vi "Encoders.vi"(10 "Reset":bool=TRUE, 11 "Enum":enum16{"Start", "Run", "End"}(ring)) -> (0 "Turning Speed":dbl, 1 "Linear Speed":dbl, 2 "RSpeed":dbl, 3 "LSpeed":dbl, 4 "LDistance":dbl, 5 "RDistance":dbl)   [LabVIEW 2014]
uses:
  <vilib>/Rock Robotics/SystemInterfaces/DIO/FPGA_DIOChannel.ctl
  <vilib>/Rock Robotics/WPI/Counter/WPI_CounterDigitalInputToDigitalSource.vi
  <vilib>/Rock Robotics/Network Tables/SD Write Number.vi
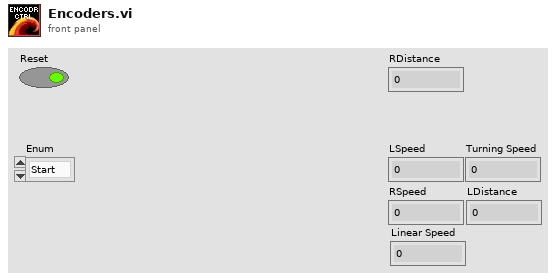
[diagram p1: front panel]
types:
  T1 = typedef "FPGA_DIOChannel.ctl" = enum8{"DIO 0", "DIO 1", "DIO 2", "DIO 3", "DIO 4", "DIO 5", "DIO 6", "DIO 7", "DIO 8", "DIO 9", "DIO MXP 0", "DIO MXP 1", "DIO MXP 2", "DIO MXP 3", "DIO MXP 4", "DIO MXP 5", "DIO MXP 6", "DIO MXP 7", "DIO MXP 8", "DIO MXP 9", "DIO MXP 10", "DIO MXP 11", "DIO MXP 12", "DIO MXP 13", "DIO MXP 14", "DIO MXP 15", "Invalid"}
  T2 = typedef "WPI_DigitalInputDevRef.ctl" = cluster{"DevStatus":errorcluster, "DIO Channel":T1, "Controller":T3}
  T3 = typedef "FPGA_TypedefDigitalModule.ctl" = enum16{"Controller 1"}
  T4 = typedef "FPGA_CounterEncoderSourceConvertionLVSourceType.ctl" = cluster{"DevStatus":errorcluster, "AnalogTriggerMode?":bool, "DigitalMode":cluster{"Controller":T3, "DIO Channel":T5}, "AnalogTriggerMode":cluster{"AnalogTriggerIndex":T6, "OutputType":T7}}
  T5 = typedef "FPGA_DIODigitalSourceChannel.ctl" = enum8{"DIO 0", "DIO 1", "DIO 2", "DIO 3", "DIO 4", "DIO 5", "DIO 6", "DIO 7", "DIO 8", "DIO 9", "DIO MXP 0", "DIO MXP 1", "DIO MXP 2", "DIO MXP 3", "DIO MXP 4", "DIO MXP 5", "DIO MXP 6", "DIO MXP 7", "DIO MXP 8", "DIO MXP 9", "DIO MXP 10", "DIO MXP 11", "DIO MXP 12", "DIO MXP 13", "DIO MXP 14", "DIO MXP 15", "Disabled"}
  T6 = typedef "FPGA_AnalogTriggerIndex.ctl" = enum8{"Trig 0", "Trig 1", "Trig 2", "Trig 3", "Trig 4", "Trig 5", "Trig 6", "Trig 7", "Invalid"}
  T7 = typedef "FPGA_AnalogTriggerOutType.ctl" = enum16{"InWindow", "TriggerState", "Rising", "Falling"}
  T8 = typedef "WPI_EncoderDevRef.ctl" = cluster{"DevStatus":errorcluster, "EncoderIndex":T9, "CounterIndex":T10, "DistancePerCount":dbl, "Decoding Type":T11}
  T9 = typedef "FPGA_EncoderIdx.ctl" = enum8{"Enc 0", "Enc 1", "Enc 2", "Enc 3", "Enc 4", "Enc 5", "Enc 6", "Enc 7", "Invalid"}
  T10 = typedef "FPGA_CounterCtrSystemIndex.ctl" = enum8{"Ctr 0", "Ctr 1", "Ctr 2", "Ctr 3", "Ctr 4", "Ctr 5", "Ctr 6", "Ctr 7", "Invalid"}
  T11 = typedef "WPI_EncoderType.ctl" = enum16{"1x", "2x", "4x"}
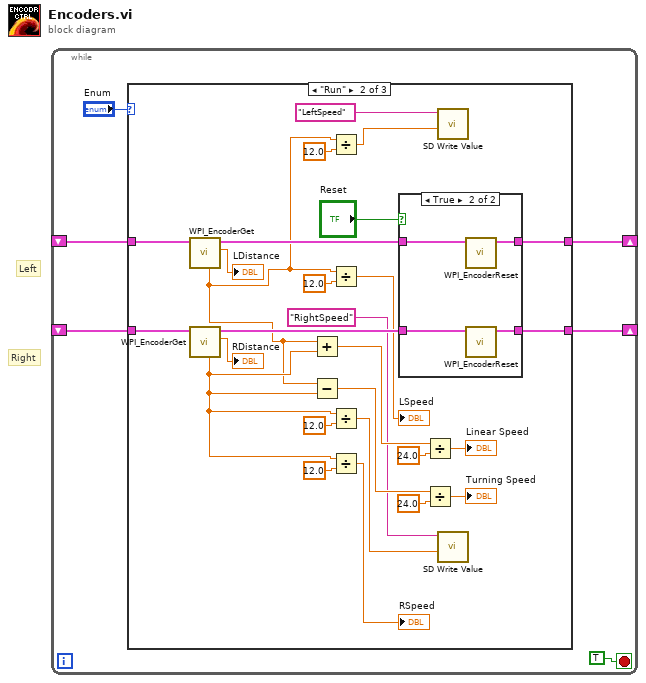
[diagram p0: block diagram]
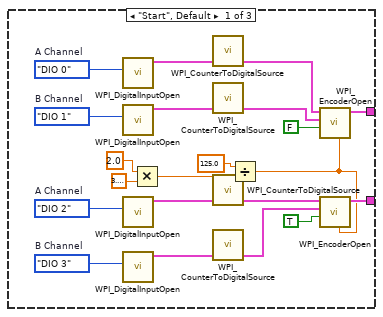
[diagram p2: hidden frame]
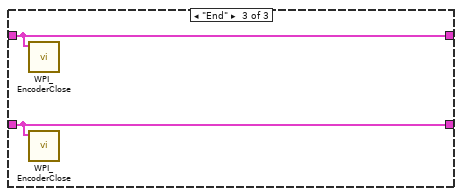
[diagram p4: hidden frame]
diagram:
  # "Right"
  # "Left"
  n1 = while {
    shift-right: [w4] -> _
    shift-left: _ -> [w2]
    shift-right: [w3] -> _
    shift-left: _ -> [w1]
    stop <- TRUE stop-if-true
    n2 = case shown="\"Run\"" "Enum" {
      tunnel: [w15 w44 w61] -> w4
      tunnel: [w14 w42 w62] -> w3
      tunnel: w2 -> [_ w54 w61]
      tunnel: w1 -> [_ w53 w62]
      frame "Start", Default {
        w21 = FPGA_DIOChannel."DIO 3"  # B Channel
        w20 = FPGA_DIOChannel."DIO 2"  # A Channel
        w27 = FPGA_DIOChannel."DIO 1"  # B Channel
        w26 = FPGA_DIOChannel."DIO 0"  # A Channel
        n3 = call <vilib>:"WPI_DigitalInputOpen.vi"("DIO Channel"=w26) -> ("DigitalInputDevRef"=w23:T2)  [unwired: 2 in, 8 out]
        n4 = call <vilib>:"WPI_DigitalInputOpen.vi"("DIO Channel"=w27) -> ("DigitalInputDevRef"=w24:T2)  [unwired: 2 in, 8 out]
        n5 = call <vilib>:"WPI_DigitalInputOpen.vi"("DIO Channel"=w20) -> ("DigitalInputDevRef"=w17:T2)  [unwired: 2 in, 8 out]
        n6 = call <vilib>:"WPI_DigitalInputOpen.vi"("DIO Channel"=w21) -> ("DigitalInputDevRef"=w18:T2)  [unwired: 2 in, 8 out]
        n7 = Multiply(x=2.0, y=3.141592653589793) -> (x*y=w9:dbl)
        n8 = call-poly <vilib>:"WPI_CounterToDigitalSource.vi"("DigitalInputDevRef"=w23) -> ("Digital Source"=w22:T4)  [unwired: 6 out]
        n9 = call-poly <vilib>:"WPI_CounterToDigitalSource.vi"("DigitalInputDevRef"=w24) -> ("Digital Source"=w25:T4)  [unwired: 6 out]
        n10 = call-poly <vilib>:"WPI_CounterToDigitalSource.vi"("DigitalInputDevRef"=w17) -> ("Digital Source"=w16:T4)  [unwired: 6 out]
        n11 = call-poly <vilib>:"WPI_CounterToDigitalSource.vi"("DigitalInputDevRef"=w18) -> ("Digital Source"=w19:T4)  [unwired: 6 out]
        n12 = Divide(x=125.0, y=w9) -> (x/y=w7:dbl)
        n13 = call <vilib>:"WPI_EncoderOpen.vi"("DistancePerCount"=w7, "Invert Direction (False)"=FALSE, "BSource"=w25, "ASource"=w22) -> ("EncoderDevRef"=w15:T8)  [unwired: 4 in, 3 out]
        n14 = call <vilib>:"WPI_EncoderOpen.vi"("DistancePerCount"=w7, "Invert Direction (False)"=TRUE, "BSource"=w19, "ASource"=w16) -> ("EncoderDevRef"=w14:T8)  [unwired: 4 in, 3 out]
      }
      frame "Run" {
        n15 = call <vilib>:"WPI_EncoderGet.vi"("EncoderDevRef"=w54) -> ("Distance"=→"LDistance":dbl, "EncoderDevRef"=w45:T8, "Rate"=w30:dbl)  [unwired: 5 in, 3 out]
        n16 = call <vilib>:"WPI_EncoderGet.vi"("EncoderDevRef"=w53) -> ("Distance"=→"RDistance":dbl, "EncoderDevRef"=w43:T8, "Rate"=w33:dbl)  [unwired: 5 in, 3 out]
        n17 = Add(x=w30, y=w33) -> (x+y=w52:dbl)
        n18 = Subtract(x=w30, y=w33) -> (x-y=w48:dbl)
        n19 = Divide(x=w30, y=12.0) -> (x/y=w28:dbl)
        n20 = Divide(x=w30, y=12.0) -> (x/y=→"LSpeed":dbl)
        n21 = Divide(x=w33, y=12.0) -> (x/y=w31:dbl)
        n22 = Divide(x=w33, y=12.0) -> (x/y=→"RSpeed":dbl)
        n23 = case shown="True" "Reset" {
          tunnel: w45 -> [w56 w60]
          tunnel: [w56 w59] -> w44
          tunnel: w43 -> [w55 w58]
          tunnel: [w55 w57] -> w42
          frame False {
          }
          frame True {
            n24 = call <vilib>:"WPI_EncoderReset.vi"("EncoderDevRef"=w60) -> ("EncoderDevRef"=w59:T8)  [unwired: 9 in, 1 out]
            n25 = call <vilib>:"WPI_EncoderReset.vi"("EncoderDevRef"=w58) -> ("EncoderDevRef"=w57:T8)  [unwired: 9 in, 1 out]
          }
        }
        n26 = Divide(x=w52, y=24.0) -> (x/y=→"Linear Speed":dbl)
        n27 = Divide(x=w48, y=24.0) -> (x/y=→"Turning Speed":dbl)
        n28 = call-poly <vilib>:"SD Write Value.vi"("Numeric"=w28, "Name"="LeftSpeed") -> ()  [unwired: 8 in, 2 out]
        n29 = call-poly <vilib>:"SD Write Value.vi"("Numeric"=w31, "Name"="RightSpeed") -> ()  [unwired: 8 in, 2 out]
      }
      frame "End" {
        n30 = call <vilib>:"WPI_EncoderClose.vi"("EncoderDevRef"=w61) -> ()  [unwired: 10 in, 1 out]
        n31 = call <vilib>:"WPI_EncoderClose.vi"("EncoderDevRef"=w62) -> ()  [unwired: 10 in, 1 out]
      }
    }
  }
